vi "Zykluszeiterfassung.vi"(6 "Aktionen":T1) -> (2 "Zykluszeiten":u32[](array[numeric]))   [LabVIEW 2020, in "allgemeine Sub-VIs.lvlib"]
uses:
  allgemeine Sub-VIs.lvlib
  Zykluszeiterfassung Aktionen.ctl
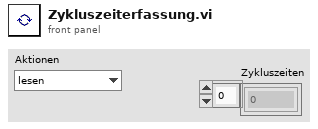
[diagram p1: front panel]
types:
  T1 = typedef "allgemeine Sub-VIs.lvlib/Zykluszeiterfassung Aktionen.ctl" = enum16{"lesen", "init", "Messdaten1", "ToolWeb", "AK FT-IR", "AK Extern", "AK Amium"}
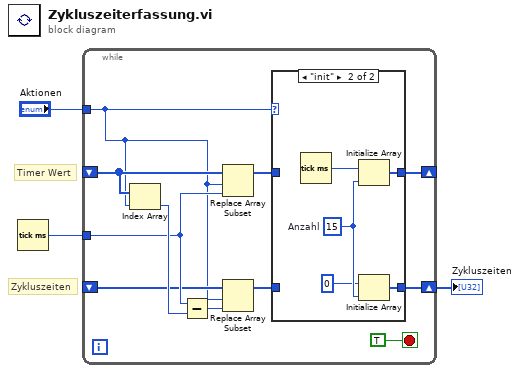
[diagram p0: block diagram]
diagram:
  # "Zykluszeiten"
  # "Timer Wert"
  n1 = Tick Count (ms)() -> (millisecond timer value=w3:u32)
  n2 = while {
    tunnel: "Aktionen" -> [w4]
    shift-right: [w13] -> _
    shift-left: _ -> [w9]
    tunnel: w3 -> [w8]
    shift-right: [w12] -> w2
    shift-left: _ -> [w7]
    stop <- TRUE stop-if-true
    n3 = Index Array(array=w9, index=w4) -> (element=w11:u32)
    n4 = Subtract(x=w8, y=w11) -> (x-y=w10:u32)
    n5 = Replace Array Subset(array=w9, new element=w8, index=w4) -> (w6:u32[])
    n6 = Replace Array Subset(array=w7, new element=w10, index=w4) -> (w5:u32[])
    n7 = case shown="\"init\"" w4 {
      tunnel: [w16 w19] -> w13
      tunnel: w6 -> [w16 _]
      tunnel: [w15 w18] -> w12
      tunnel: w5 -> [w15 _]
      frame "lesen", Default {
      }
      frame "init" {
        w21 = 15  # Anzahl
        n8 = Tick Count (ms)() -> (millisecond timer value=w20:u32)
        n9 = Initialize Array(w20, w21) -> (w19:u32[])
        n10 = Initialize Array(u32 0 ("Timer-Wert (ms)"), w21) -> (w18:u32[])
      }
    }
  }
  "Zykluszeiten" <- w2
